vi "Template Convert preV5 cluster to Keys.vi"(7 "ALL Fields":T1[](array[typedef]), 8 "error in (no error)":errorcluster, 10 "EncodedParameters":string, 11 "Old Template Record":T4) -> (0 "error out":errorcluster, 2 "(key,values)":T5, 3 "New Template Record":T4)   [LabVIEW 2011]
uses:
  DIAdem/Datasheet/Datasheet Sxx Parameters.ctl
  DIAdem/Datasheet/Datasheet Sxx Plot Formats.ctl
  DIAdem/Datasheet/Datasheet Sxx Plot Control.ctl
  DIAdem/Datasheet/Datasheet Sxx Frequency Units.ctl
  ITK EXT/utils/keyedarr.llb/Keyed Array.ctl
  Template Record.ctl
  Fields/Field Record.ctl
  Fields/Field DataTypes.ctl
  Fields/Field NextItem.ctl
  ITK EXT/utils/strutil.llb/Case Matching.ctl
panel:
  out "Report Variables":T6={"REPORT_TDR_PATH"="SXX Report", "ROOT_PATH"="", "PLOT1_TDM_PATH"="", "REPORT_PDF_PATH"="", "PLOT1_RUN_ID"=1, "PLOT_STYLE"=0, "COMPANY_ID_TXT"="", "DATETIME_TXT"="", "OPERATOR_TXT"="", "SERIALNUMBER_TXT"="", "MODELNUMBER_TXT"="", "SEQID_TXT"="", "INSTRID_TXT"="", "CUSTOMTXT 1"="", "CUSTOMTXT 2"="", "CUSTOMTXT 3"="", "CUSTOMTXT 4"="", "CUSTOMTXT 5"="", "CUSTOMTXT 6"="", "CUSTOMTXT 7"="", "CUSTOMTXT 8"="", "CUSTOMTXT 9"="", "CUSTOMTXT 10"="", "PLOT1_LABEL_TXT"="", "PLOT1_Y_TXT"="", "PLOT1_X_TXT"="", "PLOT2_LABEL_TXT"="", "PLOT2_Y_TXT"="", "PLOT2_X_TXT"="", "REPORTFOOTER"="", "PLOT1_FORMAT"=0, "PLOT1_LINETYPE"=1, "PLOT1_CURVES"=[], "PLOT1_AUTO_X"=1, "PLOT1_XMIN"=0.0, "PLOT1_XMAX"=0.0, "PLOT1_X_UNIT"=2, "PLOT1_AUTO_Y"=1, "PLOT1_YMIN"=0.0, "PLOT1_YMAX"=0.0, "PLOT2_FORMAT"=0, "PLOT2_LINETYPE"=1, "PLOT2_CURVES"=[], "PLOT2_AUTO_X"=1, "PLOT2_XMIN"=0.0, "PLOT2_XMAX"=0.0, "PLOT2_X_UNIT"=2, "PLOT2_AUTO_Y"=1, "PLOT2_YMIN"=0.0, "PLOT2_YMAX"=0.0, "PRINTER"="", "CUSTOMTXT 11"="", "CUSTOMTXT 12"="", "CUSTOMTXT 13"="", "CUSTOMTXT 14"="", "CUSTOMTXT 15"="", "CUSTOMTXT 16"="", "CUSTOMTXT 17"="", "CUSTOMTXT 18"="", "CUSTOMTXT 19"="", "CUSTOMTXT 20"="", "Custom_Count"=1, "PLOT1_MARKERS"=[], "PLOT2_MARKERS"=[], "S2P"=1, "ASCII"=1} {"PLOT2_X_UNIT" items=["Hz", "kHz", "MHz", "GHz"]; "PLOT2_FORMAT" items=["Log Magnitude", "Phase", "Delay", "Linear Magnitude", "VSWR", "Insertion Loss", "Isolation", "Return Loss", "Expanded Phase"]; "PLOT1_X_UNIT" items=["Hz", "kHz", "MHz", "GHz"]; "PLOT1_FORMAT" items=["Log Magnitude", "Phase", "Delay", "Linear Magnitude", "VSWR", "Insertion Loss", "Isolation", "Return Loss", "Expanded Phase"]; "PLOT_STYLE" items=["PDF", "HTML"]}
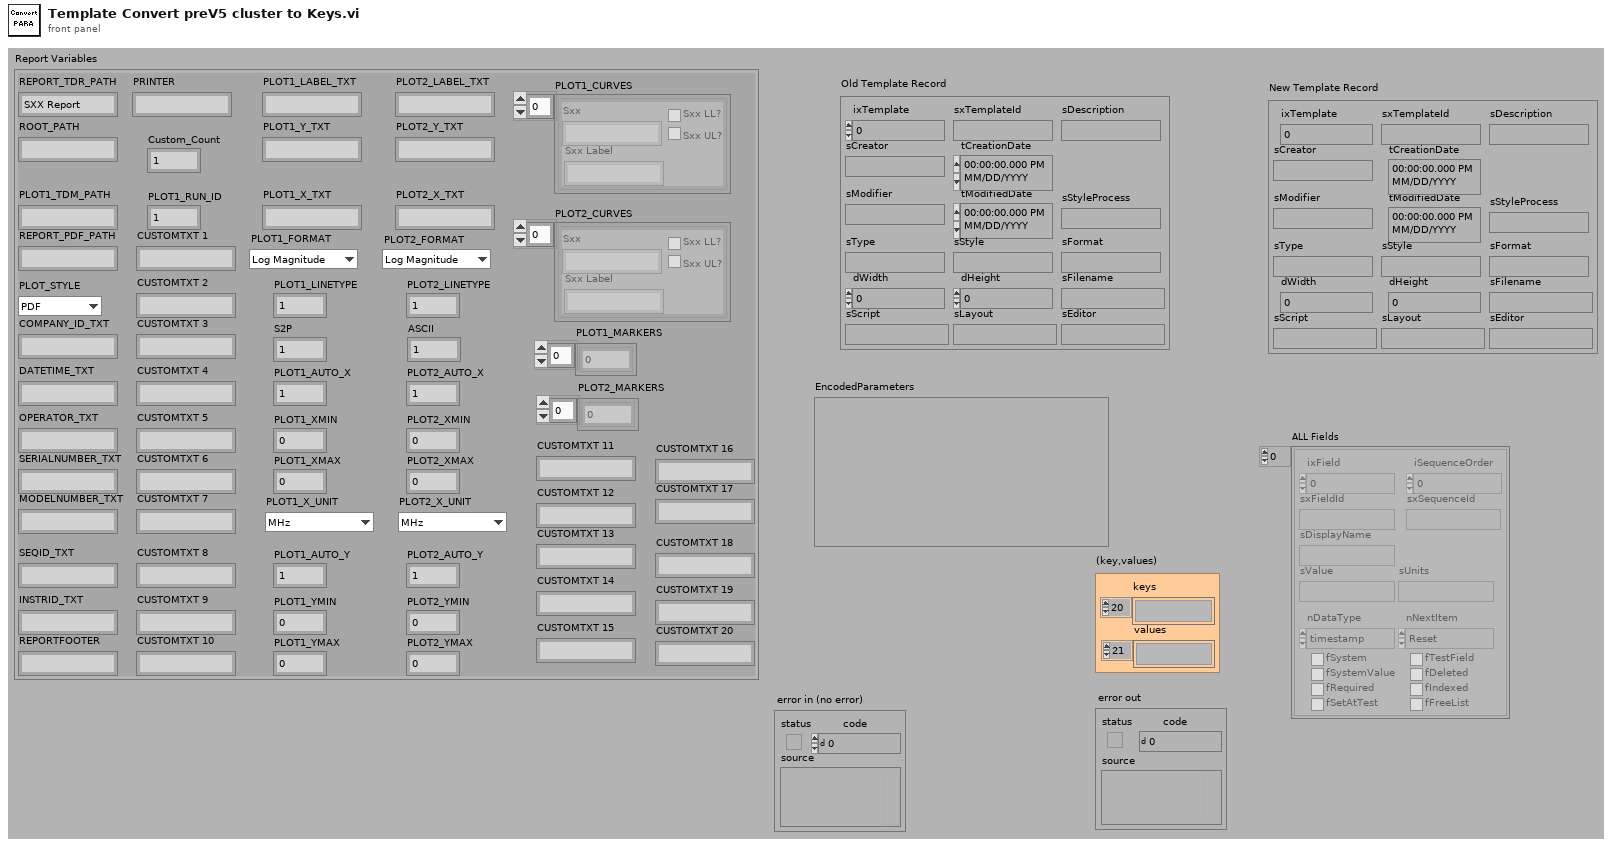
[diagram p1: front panel]
types:
  T1 = typedef "Field Record.ctl" = cluster{"ixField":i32, "iSequenceOrder":i32, "sxFieldId":string, "sxSequenceId":string, "sDisplayName":string, "sValue":string, "sUnits":string, "nDataType":T2, "nNextItem":T3, "fSystem":bool, "fSystemValue":bool, "fRequired":bool, "fSetAtTest":bool, "fTestField":bool, "fDeleted":bool, "fIndexed":bool, "fFreeList":bool}
  T2 = typedef "Field DataTypes.ctl" = enum32{"text", "numeric", "list", "timestamp", "boolean"}
  T3 = typedef "Field NextItem.ctl" = enum32{"Reset", "Retain", "Auto-Increment"}
  T4 = typedef "Template Record.ctl" = cluster{"ixTemplate":i32, "sxTemplateId":string, "sDescription":string, "sCreator":string, "tCreationDate":timestamp, "sModifier":string, "tModifiedDate":timestamp, "sType":string, "sStyle":string, "sFormat":string, "dWidth":dbl, "dHeight":dbl, "sFilename":string, "sScript":string, "sLayout":string, "sEditor":string, "sStyleProcess":string}
  T5 = typedef "Keyed Array.ctl" = cluster{"keys":string[], "values":string[]}
  T6 = typedef "DATASHEET Sxx Parameters.ctl" = cluster{"REPORT_TDR_PATH":string, "ROOT_PATH":string, "PLOT1_TDM_PATH":string, "REPORT_PDF_PATH":string, "PLOT1_RUN_ID":i32, "PLOT_STYLE":u16, "COMPANY_ID_TXT":string, "DATETIME_TXT":string, "OPERATOR_TXT":string, "SERIALNUMBER_TXT":string, "MODELNUMBER_TXT":string, "SEQID_TXT":string, "INSTRID_TXT":string, "CUSTOMTXT 1":string, "CUSTOMTXT 2":string, "CUSTOMTXT 3":string, "CUSTOMTXT 4":string, "CUSTOMTXT 5":string, "CUSTOMTXT 6":string, "CUSTOMTXT 7":string, "CUSTOMTXT 8":string, "CUSTOMTXT 9":string, "CUSTOMTXT 10":string, "PLOT1_LABEL_TXT":string, "PLOT1_Y_TXT":string, "PLOT1_X_TXT":string, "PLOT2_LABEL_TXT":string, "PLOT2_Y_TXT":string, "PLOT2_X_TXT":string, "REPORTFOOTER":string, "PLOT1_FORMAT":T7, "PLOT1_LINETYPE":i32, "PLOT1_CURVES":T8[], "PLOT1_AUTO_X":i32, "PLOT1_XMIN":dbl, "PLOT1_XMAX":dbl, "PLOT1_X_UNIT":T9, "PLOT1_AUTO_Y":i32, "PLOT1_YMIN":dbl, "PLOT1_YMAX":dbl, "PLOT2_FORMAT":T7, "PLOT2_LINETYPE":i32, "PLOT2_CURVES":T8[], "PLOT2_AUTO_X":i32, "PLOT2_XMIN":dbl, "PLOT2_XMAX":dbl, "PLOT2_X_UNIT":T9, "PLOT2_AUTO_Y":i32, "PLOT2_YMIN":dbl, "PLOT2_YMAX":dbl, "PRINTER":string, "CUSTOMTXT 11":string, "CUSTOMTXT 12":string, "CUSTOMTXT 13":string, "CUSTOMTXT 14":string, "CUSTOMTXT 15":string, "CUSTOMTXT 16":string, "CUSTOMTXT 17":string, "CUSTOMTXT 18":string, "CUSTOMTXT 19":string, "CUSTOMTXT 20":string, "Custom_Count":i32, "PLOT1_MARKERS":dbl[], "PLOT2_MARKERS":dbl[], "S2P":i32, "ASCII":i32}
  T7 = typedef "DATASHEET Sxx Plot Formats.ctl" = u16
  T8 = typedef "DATASHEET Sxx Plot Control.ctl" = cluster{"Sxx":string, "Sxx LL?":bool, "Sxx UL?":bool, "Sxx Label":string}
  T9 = typedef "DATASHEET Sxx Frequency Units.ctl" = u16
  T10 = typedef "Case Matching.ctl" = enum16{"a != A", "a == A", "system"}
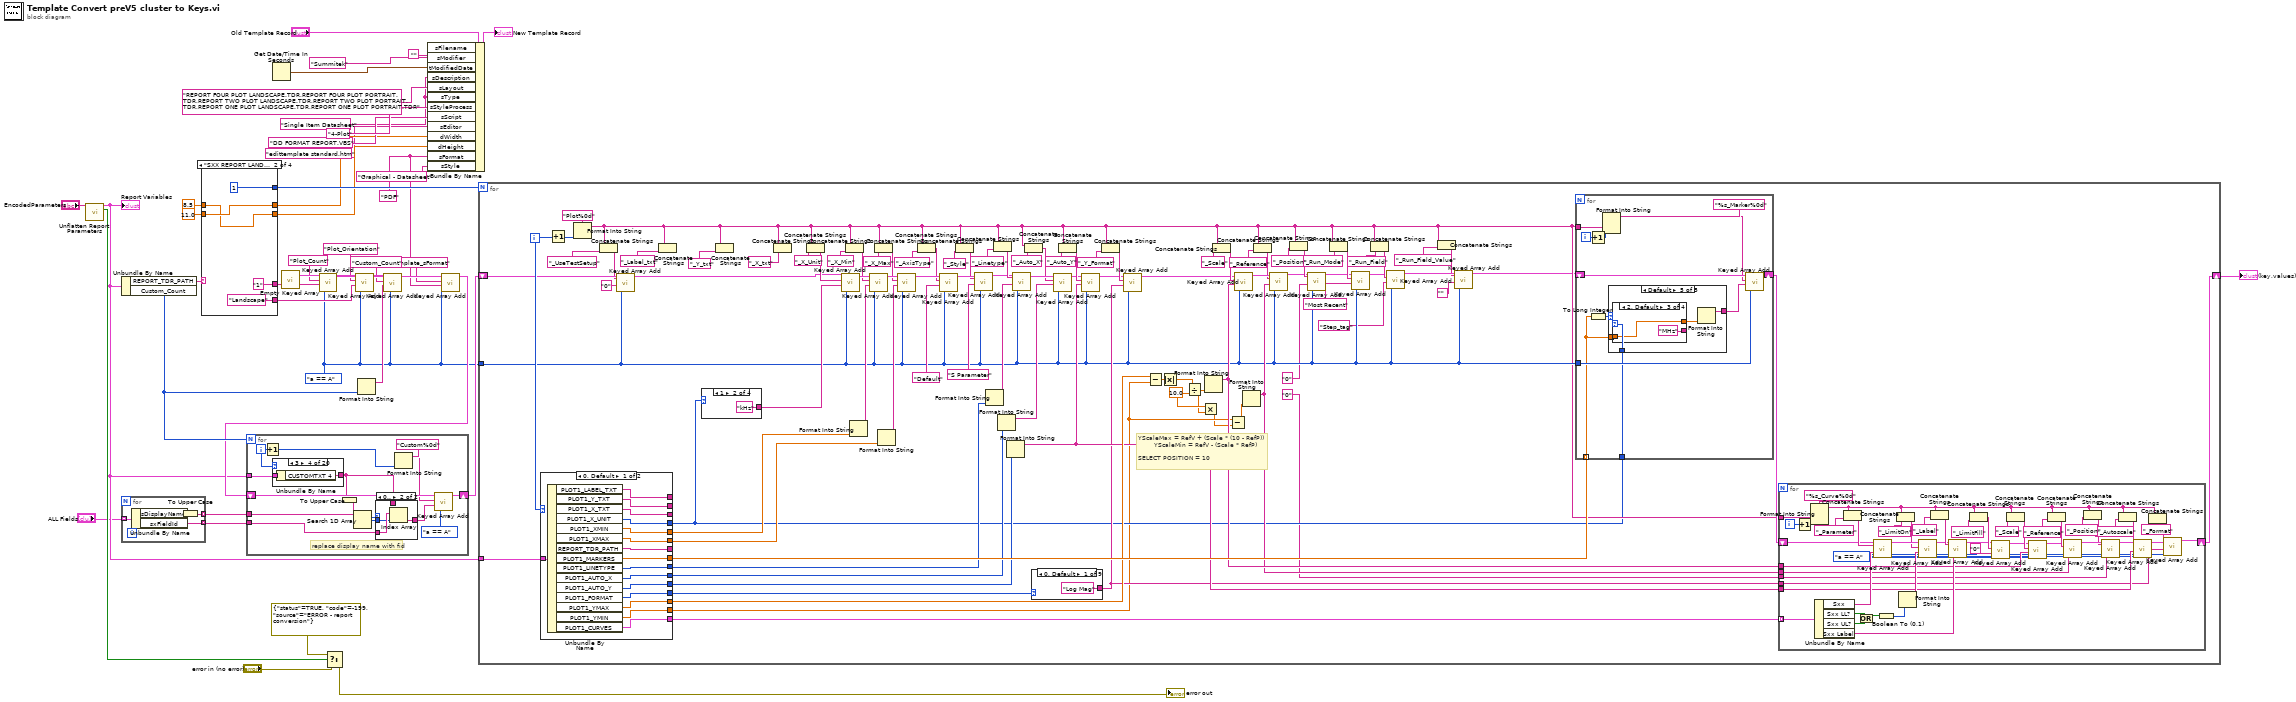
[diagram p0: block diagram]
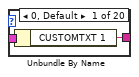
[diagram p3: hidden frame]
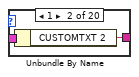
[diagram p4: hidden frame]
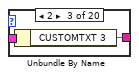
[diagram p5: hidden frame]
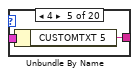
[diagram p6: hidden frame]
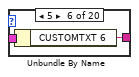
[diagram p7: hidden frame]
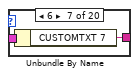
[diagram p8: hidden frame]
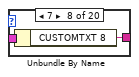
[diagram p9: hidden frame]
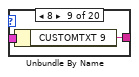
[diagram p10: hidden frame]
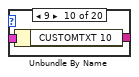
[diagram p11: hidden frame]
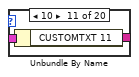
[diagram p12: hidden frame]
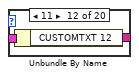
[diagram p13: hidden frame]
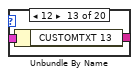
[diagram p14: hidden frame]
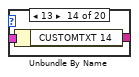
[diagram p15: hidden frame]
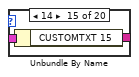
[diagram p16: hidden frame]
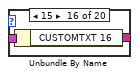
[diagram p17: hidden frame]
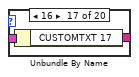
[diagram p18: hidden frame]
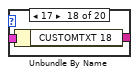
[diagram p19: hidden frame]
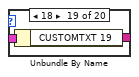
[diagram p20: hidden frame]
diagram:
  w8 = "PDF" ("sType")
  w5 = "Single Item Datasheet" ("sType")
  w26 = Case_Matching."a == A" ("case matching (sensitive)")
  n1 = call "Unflatten Report Parameters.vi"("Parameter String"="EncodedParameters") -> ("Error"=w23:bool, "Report Parameters"=w24:T6)  [unwired: 9 out]
  "Report Variables" <- w24
  n2 = Unbundle By Name(w24) -> ("REPORT_TDR_PATH"=w43:string, "Custom_Count"=w31:i32)
  n3 = for {
    tunnel: "ALL Fields" -> [w47] mode=indexing
    tunnel: [w44] -> w14 mode=indexing
    tunnel: [w45] -> w13 mode=indexing
    n4 = Unbundle By Name(w47) -> ("sDisplayName"=w46:string, "sxFieldId"=w45:string)
    n5 = To Upper Case(1:w46) -> (0:w44:string)
  }
  n6 = case shown="\"SXX REPORT LANDSCAPE.TDR\"" w43 {
    tunnel: ["1" ("sxFieldId") "1" ("sxFieldId") "2" ("sxFieldId") "2" ("sxFieldId")] -> w40
    tunnel: ["Portrait" ("sxFieldId") "Landscape" ("sxFieldId") "Portrait" ("sxFieldId") "Landscape" ("sxFieldId")] -> w37
    tunnel: [1 1 2 2] -> w30
    tunnel: [w49 w54 w59 w64] -> w12
    tunnel: [w48 w53 w58 w63] -> w11
    tunnel: 8.5 ("dWidth") -> [w49 w53 w59 w63]
    tunnel: 11.0 ("dHeight") -> [w48 w54 w58 w64]
    frame "SXX REPORT.TDR", Default {
    }
    frame "SXX REPORT LANDSCAPE.TDR" {
    }
    frame "SXX REPORT TWO PLOT.TDR" {
    }
    frame "SXX REPORT TWO PLOT LANDSCAPE.TDR" {
    }
  }
  n7 = Get Date/Time In Seconds() -> (seconds since 1Jan1904=w2:timestamp)
  n8 = call "Empty Keyed Array.vi"() -> ("empty keyed array"=w42:T5)  [unwired: 3 out]
  n9 = call "Keyed Array Add.vi"("case matching (sensitive)"=w26, "value"=w40, "key"="Plot_Count" ("sxFieldId"), "array in"=w42) -> ("array out"=w39:T5)  [unwired: 3 out]
  n10 = Select(t=errorcluster {"status"=TRUE, "code"=-199, "source"="ERROR - report conversion"}, s=w23, f="error in (no error)") -> (s? t:f=→"error out":errorcluster)
  n11 = call "Keyed Array Add.vi"("case matching (sensitive)"=w26, "value"=w37, "key"="Plot_Orientation" ("sxFieldId"), "array in"=w39) -> ("array out"=w34:T5)  [unwired: 3 out]
  n12 = Format Into String(w31) -> (resulting string=w32:string)  [unwired: 3 in, 1 out]
  n13 = call "Keyed Array Add.vi"("case matching (sensitive)"=w26, "value"=w32, "key"="Custom_Count" ("sxFieldId"), "array in"=w34) -> ("array out"=w29:T5)  [unwired: 3 out]
  n14 = Bundle By Name(cluster="Old Template Record", "sFilename"="", "sModifier"="Summitek" ("sType"), "tModifiedDate"=w2, "sDescription"=w5, "sLayout"="REPORT FOUR PLOT LANDSCAPE.TDR,REPORT FOUR PLOT PORTRAIT.TDR,REPORT TWO PLOT LANDSCAPE.TDR,REPORT TWO PLOT PORTRAIT.TDR,REPORT ONE PLOT LANDSCAPE.TDR,REPORT ONE PLOT PORTRAIT.TDR" ("sType"), "sType"=w5, "sStyleProcess"="4-Plot" ("sStyle"), "sScript"="DD FORMAT REPORT.VBS", "sEditor"="edittemplate standard.htm" ("sScript"), "dWidth"=w12, "dHeight"=w11, "sFormat"=w8, "sStyle"="Graphical - Datasheet") -> (→"New Template Record":T4)
  n15 = call "Keyed Array Add.vi"("case matching (sensitive)"=w26, "value"=w8, "key"="Template_sFormat" ("sxFieldId"), "array in"=w29) -> ("array out"=w28:T5)  [unwired: 3 out]
  n16 = for {
    N: w31 -> [_]
    shift-right: [w78] -> w35
    shift-left: w28 -> [w79]
    tunnel: w24 -> [w75]
    tunnel: w14 -> [w73]
    tunnel: w13 -> [w72]
    i -> [w76]
    # "replace display name with fid"
    n17 = Increment(x=w76) -> (x+1=w80:i32)
    n18 = case shown="3" w76 {
      tunnel: [w87 w89 w91 w93 w95 w97 w99 w101 w103 w105 w107 w109 w111 w113 w115 w117 w119 w121 w123 w125] -> w68
      tunnel: w75 -> [w86 w88 w90 w92 w94 w96 w98 w100 w102 w104 w106 w108 w110 w112 w114 w116 w118 w120 w122 w124]
      frame 0, Default {
        n19 = Unbundle By Name(w86) -> ("CUSTOMTXT 1"=w87:string)
      }
      frame 1 {
        n20 = Unbundle By Name(w88) -> ("CUSTOMTXT 2"=w89:string)
      }
      frame 2 {
        n21 = Unbundle By Name(w90) -> ("CUSTOMTXT 3"=w91:string)
      }
      frame 3 {
        n22 = Unbundle By Name(w92) -> ("CUSTOMTXT 4"=w93:string)
      }
      frame 4 {
        n23 = Unbundle By Name(w94) -> ("CUSTOMTXT 5"=w95:string)
      }
      frame 5 {
        n24 = Unbundle By Name(w96) -> ("CUSTOMTXT 6"=w97:string)
      }
      frame 6 {
        n25 = Unbundle By Name(w98) -> ("CUSTOMTXT 7"=w99:string)
      }
      frame 7 {
        n26 = Unbundle By Name(w100) -> ("CUSTOMTXT 8"=w101:string)
      }
      frame 8 {
        n27 = Unbundle By Name(w102) -> ("CUSTOMTXT 9"=w103:string)
      }
      frame 9 {
        n28 = Unbundle By Name(w104) -> ("CUSTOMTXT 10"=w105:string)
      }
      frame 10 {
        n29 = Unbundle By Name(w106) -> ("CUSTOMTXT 11"=w107:string)
      }
      frame 11 {
        n30 = Unbundle By Name(w108) -> ("CUSTOMTXT 12"=w109:string)
      }
      frame 12 {
        n31 = Unbundle By Name(w110) -> ("CUSTOMTXT 13"=w111:string)
      }
      frame 13 {
        n32 = Unbundle By Name(w112) -> ("CUSTOMTXT 14"=w113:string)
      }
      frame 14 {
        n33 = Unbundle By Name(w114) -> ("CUSTOMTXT 15"=w115:string)
      }
      frame 15 {
        n34 = Unbundle By Name(w116) -> ("CUSTOMTXT 16"=w117:string)
      }
      frame 16 {
        n35 = Unbundle By Name(w118) -> ("CUSTOMTXT 17"=w119:string)
      }
      frame 17 {
        n36 = Unbundle By Name(w120) -> ("CUSTOMTXT 18"=w121:string)
      }
      frame 18 {
        n37 = Unbundle By Name(w122) -> ("CUSTOMTXT 19"=w123:string)
      }
      frame 19 {
        n38 = Unbundle By Name(w124) -> ("CUSTOMTXT 20"=w125:string)
      }
    }
    n39 = To Upper Case(1:w68) -> (0:w71:string)
    n40 = Search 1D Array(1D array=w73, element=w71) -> (index of element=w69:i32)  [unwired: 1 out]
    n41 = case shown="0.." w69 {
      tunnel: w72 -> [_ w85]
      tunnel: w69 -> [_ w84]
      tunnel: [w82 w83] -> w70
      tunnel: w68 -> [w82 _]
      frame Default {
      }
      frame 0.. {
        n42 = Index Array(array=w85, index=w84) -> (element=w83:string)
      }
    }
    n43 = Format Into String(format string="Custom%0d" ("sxFieldId"), w80) -> (resulting string=w77:string)  [unwired: 2 in, 1 out]
    n44 = call "Keyed Array Add.vi"("case matching (sensitive)"=Case_Matching."a == A", "value"=w70, "key"=w77, "array in"=w79) -> ("array out"=w78:T5)  [unwired: 3 out]
  }
  n45 = for {
    N: w30 -> [_]
    tunnel: w24 -> [w219]
    shift-right: [w158] -> w36
    shift-left: w35 -> [w200]
    tunnel: w26 -> [w141]
    i -> [w201]
    w130 = 10.0 ("y")
    # "YScaleMax = RefV + (Scale * (10 - RefP))\n        YScaleMin = RefV - (Scale * RefP)\n\nSELECT POSITION = 10"
    n46 = case shown="0, Default" w201 {
      tunnel: w219 -> [w248 w264]
      tunnel: [w247 w263] -> w133
      tunnel: [w246 w262] -> w214
      tunnel: [w245 w261] -> w213
      tunnel: [w244 w260] -> _
      tunnel: [w243 w259] -> w211
      tunnel: [w242 w258] -> _
      tunnel: [w241 w257] -> _
      tunnel: [w240 w256] -> _
      tunnel: [w239 w255] -> w186
      tunnel: [w238 w254] -> w175
      tunnel: [w237 w253] -> w173
      tunnel: [w236 w252] -> w170
      tunnel: [w235 w251] -> w161
      tunnel: [w234 w250] -> w128
      tunnel: [w233 w249] -> w157
      frame 0, Default {
        n47 = Unbundle By Name(w248) -> ("PLOT1_LABEL_TXT"=w242:string, "PLOT1_Y_TXT"=w241:string, "PLOT1_X_TXT"=w240:string, "PLOT1_X_UNIT"=w247:T9, "PLOT1_XMIN"=w246:dbl, "PLOT1_XMAX"=w245:dbl, "REPORT_TDR_PATH"=w244:string, "PLOT1_MARKERS"=w243:dbl[], "PLOT1_LINETYPE"=w239:i32, "PLOT1_AUTO_X"=w238:i32, "PLOT1_AUTO_Y"=w237:i32, "PLOT1_FORMAT"=w236:T7, "PLOT1_YMAX"=w235:dbl, "PLOT1_YMIN"=w234:dbl, "PLOT1_CURVES"=w233:T8[])
      }
      frame 1 {
        n48 = Unbundle By Name(w264) -> ("PLOT2_LABEL_TXT"=w258:string, "PLOT2_Y_TXT"=w257:string, "PLOT2_X_TXT"=w256:string, "PLOT2_X_UNIT"=w263:T9, "PLOT2_XMIN"=w262:dbl, "PLOT2_XMAX"=w261:dbl, "REPORT_TDR_PATH"=w260:string, "PLOT2_MARKERS"=w259:dbl[], "PLOT2_LINETYPE"=w255:i32, "PLOT2_AUTO_X"=w254:i32, "PLOT2_AUTO_Y"=w253:i32, "PLOT2_FORMAT"=w252:T7, "PLOT2_XMAX"=w251:dbl, "PLOT2_YMIN"=w250:dbl, "PLOT2_CURVES"=w249:T8[])
      }
    }
    n49 = Increment(x=w201) -> (x+1=w210:i32)
    n50 = Format Into String(format string="Plot%0d" ("sxFieldId"), w210) -> (resulting string=w137:string)  [unwired: 2 in, 1 out]
    n51 = Concatenate Strings(w137, "_UseTestSetup" ("sxFieldId")) -> (w198:string)
    n52 = call "Keyed Array Add.vi"("case matching (sensitive)"=w141, "value"="0", "key"=w198, "array in"=w200) -> ("array out"=w136:T5)  [unwired: 3 out]
    n53 = Concatenate Strings(w137, "_Label_txt" ("sxFieldId")) -> ()  [unwired: 1 out]
    n54 = case shown="1" w133 {
      tunnel: ["Hz" ("sxFieldId") "kHz" ("sxFieldId") "MHz" ("sxFieldId") "GHz" ("sxFieldId")] -> w172
      frame 0 {
      }
      frame 1 {
      }
      frame 2, Default {
      }
      frame 3 {
      }
    }
    n55 = Concatenate Strings(w137, "_Y_txt" ("sxFieldId")) -> ()  [unwired: 1 out]
    n56 = Concatenate Strings(w137, "_X_txt" ("sxFieldId")) -> ()  [unwired: 1 out]
    n57 = Concatenate Strings(w137, "_X_Unit" ("sxFieldId")) -> (w209:string)
    n58 = call "Keyed Array Add.vi"("case matching (sensitive)"=w141, "value"=w172, "key"=w209, "array in"=w136) -> ("array out"=w208:T5)  [unwired: 3 out]
    n59 = Concatenate Strings(w137, "_X_Min" ("sxFieldId")) -> (w207:string)
    n60 = Format Into String(w214) -> (resulting string=w206:string)  [unwired: 3 in, 1 out]
    n61 = call "Keyed Array Add.vi"("case matching (sensitive)"=w141, "value"=w206, "key"=w207, "array in"=w208) -> ("array out"=w205:T5)  [unwired: 3 out]
    n62 = Concatenate Strings(w137, "_X_Max" ("sxFieldId")) -> (w204:string)
    n63 = Format Into String(w213) -> (resulting string=w203:string)  [unwired: 3 in, 1 out]
    n64 = call "Keyed Array Add.vi"("case matching (sensitive)"=w141, "value"=w203, "key"=w204, "array in"=w205) -> ("array out"=w202:T5)  [unwired: 3 out]
    n65 = Concatenate Strings(w137, "_AxisType" ("sxFieldId")) -> (w194:string)
    n66 = call "Keyed Array Add.vi"("case matching (sensitive)"=w141, "value"="Default" ("sxFieldId"), "key"=w194, "array in"=w202) -> ("array out"=w193:T5)  [unwired: 3 out]
    n67 = Concatenate Strings(w137, "_Style" ("sxFieldId")) -> (w191:string)
    n68 = call "Keyed Array Add.vi"("case matching (sensitive)"=w141, "value"="S Parameter" ("sxFieldId"), "key"=w191, "array in"=w193) -> ("array out"=w188:T5)  [unwired: 3 out]
    n69 = Format Into String(w186) -> (resulting string=w185:string)  [unwired: 3 in, 1 out]
    n70 = Concatenate Strings(w137, "_Linetype" ("sxFieldId")) -> (w189:string)
    n71 = Format Into String(w175) -> (resulting string=w174:string)  [unwired: 3 in, 1 out]
    n72 = Format Into String(w173) -> (resulting string=w152:string)  [unwired: 3 in, 1 out]
    n73 = call "Keyed Array Add.vi"("case matching (sensitive)"=w141, "value"=w185, "key"=w189, "array in"=w188) -> ("array out"=w178:T5)  [unwired: 3 out]
    n74 = Concatenate Strings(w137, "_Auto_X" ("sxFieldId")) -> (w176:string)
    n75 = case shown="0, Default" w170 {
      tunnel: ["Log Mag" ("sxFieldId") "Phase" ("sxFieldId") "Delay" ("sxFieldId") "Lin Mag" ("sxFieldId") "SWR" ("sxFieldId") "Loss" ("sxFieldId") "Loss" ("sxFieldId") "Loss" ("sxFieldId") "Expanded Phase" ("sxFieldId")] -> w151
      frame 0, Default {
      }
      frame 1 {
      }
      frame 2 {
      }
      frame 3 {
      }
      frame 4 {
      }
      frame 5 {
      }
      frame 6 {
      }
      frame 7 {
      }
      frame 8 {
      }
    }
    n76 = call "Keyed Array Add.vi"("case matching (sensitive)"=w141, "value"=w174, "key"=w176, "array in"=w178) -> ("array out"=w181:T5)  [unwired: 3 out]
    n77 = Concatenate Strings(w137, "_Auto_Y" ("sxFieldId")) -> (w182:string)
    n78 = call "Keyed Array Add.vi"("case matching (sensitive)"=w141, "value"=w152, "key"=w182, "array in"=w181) -> ("array out"=w183:T5)  [unwired: 3 out]
    n79 = Concatenate Strings(w137, "_Y_Format" ("sxFieldId")) -> (w184:string)
    n80 = call "Keyed Array Add.vi"("case matching (sensitive)"=w141, "value"=w151, "key"=w184, "array in"=w183) -> ("array out"=w153:T5)  [unwired: 3 out]
    n81 = Subtract(x=w161, y=w128) -> (x-y=w160:dbl)
    n82 = Absolute Value(x=w160) -> (abs(x)=w134:dbl)
    n83 = Divide(x=w134, y=w130) -> (x/y=w129:dbl)
    n84 = Multiply(x=w130, y=w129) -> (x*y=w127:dbl)
    n85 = Format Into String(w129) -> (resulting string=w155:string)  [unwired: 3 in, 1 out]
    n86 = Concatenate Strings(w137, "_Scale" ("sxFieldId")) -> (w169:string)
    n87 = Subtract(x=w128, y=w127) -> (x-y=w126:dbl)
    n88 = call "Keyed Array Add.vi"("case matching (sensitive)"=w141, "value"=w155, "key"=w169, "array in"=w153) -> ("array out"=w168:T5)  [unwired: 3 out]
    n89 = Format Into String(w126) -> (resulting string=w154:string)  [unwired: 3 in, 1 out]
    n90 = Concatenate Strings(w137, "_Reference" ("sxFieldId")) -> (w166:string)
    n91 = call "Keyed Array Add.vi"("case matching (sensitive)"=w141, "value"=w154, "key"=w166, "array in"=w168) -> ("array out"=w164:T5)  [unwired: 3 out]
    n92 = Concatenate Strings(w137, "_Position" ("sxFieldId")) -> (w165:string)
    n93 = call "Keyed Array Add.vi"("case matching (sensitive)"=w141, "value"="0" ("sxFieldId"), "key"=w165, "array in"=w164) -> ("array out"=w142:T5)  [unwired: 3 out]
    n94 = Concatenate Strings(w137, "_Run_Mode" ("sxFieldId")) -> (w143:string)
    n95 = call "Keyed Array Add.vi"("case matching (sensitive)"=w141, "value"="Most Recent" ("sxFieldId"), "key"=w143, "array in"=w142) -> ("array out"=w144:T5)  [unwired: 3 out]
    n96 = Concatenate Strings(w137, "_Run_Field" ("sxFieldId")) -> (w146:string)
    n97 = call "Keyed Array Add.vi"("case matching (sensitive)"=w141, "value"="Step_tag" ("sxFieldId"), "key"=w146, "array in"=w144) -> ("array out"=w148:T5)  [unwired: 3 out]
    n98 = Concatenate Strings(w137, "_Run_Field_Value" ("sxFieldId")) -> (w147:string)
    n99 = call "Keyed Array Add.vi"("case matching (sensitive)"=w141, "value"="", "key"=w147, "array in"=w148) -> ("array out"=w135:T5)  [unwired: 3 out]
    n100 = for {
      tunnel: w211 -> [w316] mode=indexing
      tunnel: w137 -> [w323]
      shift-right: [w319] -> w159
      shift-left: w135 -> [w320]
      tunnel: w141 -> [w317]
      tunnel: w133 -> [w313]
      i -> [w322]
      n101 = Increment(x=w322) -> (x+1=w321:i32)
      n102 = To Long Integer(number=w316) -> (32bit integer=w314:i32)
      n103 = Format Into String(format string="%s_Marker%0d" ("sxFieldId"), w323, w321) -> (resulting string=w318:string)  [unwired: 2 in, 1 out]
      n104 = case shown="Default" w314 {
        tunnel: w316 -> [_ _ _ _ w330]
        tunnel: ["Trace Maximum" "Trace Minimum" "Limit Maximum" "Limit Minimum" w332] -> w315
        tunnel: w313 -> [_ _ _ _ w331]
        frame -1 {
        }
        frame -2 {
        }
        frame -3 {
        }
        frame -4 {
        }
        frame Default {
          n105 = case shown="2, Default" w331 {
            tunnel: ["Hz" ("sxFieldId") "kHz" ("sxFieldId") "MHz" ("sxFieldId") "GHz" ("sxFieldId")] -> _
            tunnel: w330 -> [w334 w338 w341 w345]
            tunnel: [w335 w339 w341 w344] -> w329
            frame 0 {
              n106 = Multiply(x=w334, y=1000000.0) -> (x*y=w335:dbl)
            }
            frame 1 {
              n107 = Multiply(x=w338, y=1000.0) -> (x*y=w339:dbl)
            }
            frame 2, Default {
            }
            frame 3 {
              n108 = Divide(x=w345, y=1000.0) -> (x/y=w344:dbl)
            }
          }
          n109 = Format Into String(w329) -> (resulting string=w332:string)  [unwired: 3 in, 1 out]
        }
      }
      n110 = call "Keyed Array Add.vi"("case matching (sensitive)"=w317, "value"=w315, "key"=w318, "array in"=w320) -> ("array out"=w319:T5)  [unwired: 3 out]
    }
    n111 = for {
      shift-right: [w270] -> w158
      shift-left: w159 -> [w299]
      tunnel: w137 -> [w303]
      tunnel: w157 -> [w302] mode=indexing
      tunnel: w155 -> [w284]
      tunnel: w154 -> [w283]
      tunnel: "0" ("sxFieldId") -> [w282]
      tunnel: w152 -> [w267]
      tunnel: w151 -> [w265]
      i -> [w311]
      w266 = Case_Matching."a == A" ("case matching (sensitive)")
      n112 = Increment(x=w311) -> (x+1=w310:i32)
      n113 = Format Into String(format string="%s_Curve%0d" ("sxFieldId"), w303, w310) -> (resulting string=w275:string)  [unwired: 2 in, 1 out]
      n114 = Unbundle By Name(w302) -> ("Sxx"=w300:string, "Sxx LL?"=w279:bool, "Sxx UL?"=w278:bool, "Sxx Label"=w298:string)
      n115 = Concatenate Strings(w275, "_Parameter" ("sxFieldId")) -> (w304:string)
      n116 = Or(x=w279, y=w278) -> (x .or. y?=w277:bool)
      n117 = call "Keyed Array Add.vi"("case matching (sensitive)"=w266, "value"=w300, "key"=w304, "array in"=w299) -> ("array out"=w308:T5)  [unwired: 3 out]
      n118 = Boolean To (0,1)(Boolean=w277) -> (0, 1=w296:i16)
      n119 = Concatenate Strings(w275, "_LimitOn" ("sxFieldId")) -> (w305:string)
      n120 = Format Into String(w296) -> (resulting string=w297:string)  [unwired: 3 in, 1 out]
      n121 = call "Keyed Array Add.vi"("case matching (sensitive)"=w266, "value"=w297, "key"=w305, "array in"=w308) -> ("array out"=w280:T5)  [unwired: 3 out]
      n122 = Concatenate Strings(w275, "_Label" ("sxFieldId")) -> (w306:string)
      n123 = call "Keyed Array Add.vi"("case matching (sensitive)"=w266, "value"=w298, "key"=w306, "array in"=w280) -> ("array out"=w286:T5)  [unwired: 3 out]
      n124 = Concatenate Strings(w275, "_LimitFill" ("sxFieldId")) -> (w287:string)
      n125 = call "Keyed Array Add.vi"("case matching (sensitive)"=w266, "value"="0" ("sxFieldId"), "key"=w287, "array in"=w286) -> ("array out"=w276:T5)  [unwired: 3 out]
      n126 = Concatenate Strings(w275, "_Scale" ("sxFieldId")) -> (w288:string)
      n127 = call "Keyed Array Add.vi"("case matching (sensitive)"=w266, "value"=w284, "key"=w288, "array in"=w276) -> ("array out"=w289:T5)  [unwired: 3 out]
      n128 = Concatenate Strings(w275, "_Reference" ("sxFieldId")) -> (w291:string)
      n129 = call "Keyed Array Add.vi"("case matching (sensitive)"=w266, "value"=w283, "key"=w291, "array in"=w289) -> ("array out"=w293:T5)  [unwired: 3 out]
      n130 = Concatenate Strings(w275, "_Position" ("sxFieldId")) -> (w292:string)
      n131 = call "Keyed Array Add.vi"("case matching (sensitive)"=w266, "value"=w282, "key"=w292, "array in"=w293) -> ("array out"=w272:T5)  [unwired: 3 out]
      n132 = Concatenate Strings(w275, "_Autoscale" ("sxFieldId")) -> (w273:string)
      n133 = call "Keyed Array Add.vi"("case matching (sensitive)"=w266, "value"=w267, "key"=w273, "array in"=w272) -> ("array out"=w271:T5)  [unwired: 3 out]
      n134 = Concatenate Strings(w275, "_Format" ("sxFieldId")) -> (w268:string)
      n135 = call "Keyed Array Add.vi"("case matching (sensitive)"=w266, "value"=w265, "key"=w268, "array in"=w271) -> ("array out"=w270:T5)  [unwired: 3 out]
    }
  }
  "(key,values)" <- w36
